vi "Unix时间截ms.vi"() -> (0 "Unix时间截ms":u64)   [LabVIEW 2017]
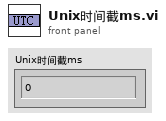
[diagram p1: front panel]
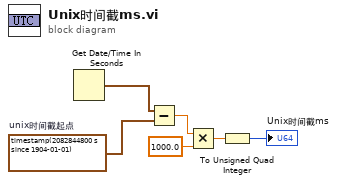
[diagram p0: block diagram]
diagram:
  w6 = timestamp(2082844800 s since 1904-01-01)  # unix时间截起点
  n1 = Get Date/Time In Seconds() -> (seconds since 1Jan1904=w1:timestamp)
  n2 = Subtract(x=w1, y=w6) -> (x-y=w3:dbl)
  n3 = Multiply(x=w3, y=1000.0) -> (x*y=w4:dbl)
  n4 = To Unsigned Quad Integer(1:w4) -> (0:→"Unix时间截ms":u64)
